vi "Error Converter (ErrCode or Status).vi"(8 "error in (no error)":errorcluster, 11 "error code":i32) -> (0 "error out":errorcluster)   [LabVIEW 2013, in "TimeTagLV.lvlib"]
uses:
  TimeTagLV.lvlib
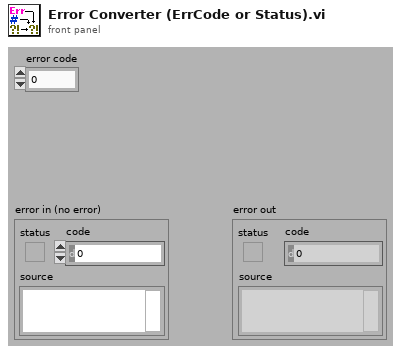
[diagram p1: front panel]
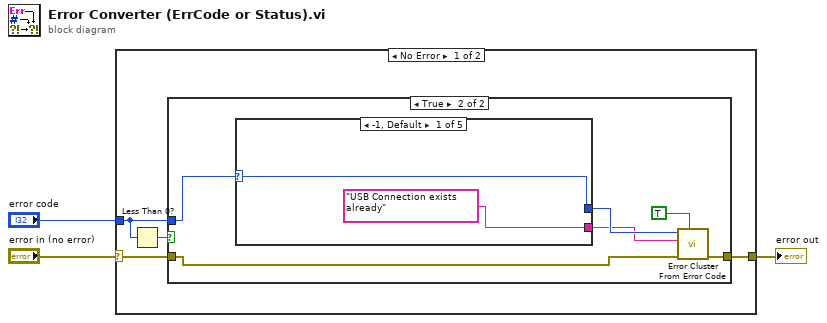
[diagram p0: block diagram]
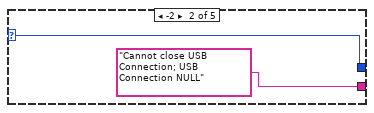
[diagram p3: hidden frame]
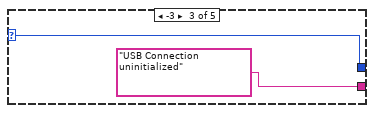
[diagram p4: hidden frame]
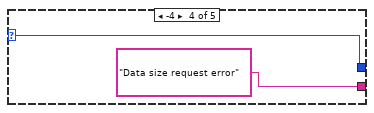
[diagram p5: hidden frame]
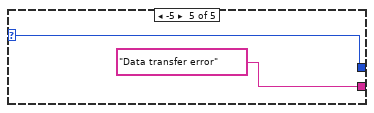
[diagram p6: hidden frame]
diagram:
  n1 = case shown="No Error" "error in (no error)" {
    selector: "error in (no error)" -> [w6 w25]
    tunnel: [w4 w25] -> w2
    tunnel: "error code" -> [w5 _]
    frame No Error {
      n2 = Less Than 0?(x=w5) -> (x < 0?=w7:bool)
      n3 = case shown="True" w7 {
        tunnel: w6 -> [w8 w11]
        tunnel: w5 -> [_ w12]
        tunnel: [w8 w14] -> w4
        frame False {
        }
        frame True {
          n4 = case shown="-1, Default" w12 {
            selector: w12 -> [w16 w18 w20 w22 w24]
            tunnel: [w16 w18 w20 w22 w24] -> w10
            tunnel: ["USB Connection exists already" "Cannot close USB Connection; USB Connection NULL" "USB Connection uninitialized" "Data size request error" "Data transfer error"] -> w9
            frame -1, Default {
            }
            frame -2 {
            }
            frame -3 {
            }
            frame -4 {
            }
            frame -5 {
            }
          }
          n5 = call <vilib>:"Error Cluster From Error Code.vi"("show call chain? (False)"=TRUE, "error in (no error)"=w11, "error message (\"\")"=w9, "error code (0)"=w10) -> ("error out"=w14:errorcluster)  [unwired: 5 in]
        }
      }
    }
    frame Error {
    }
  }
  "error out" <- w2
